vi "Write Pin.vi"(0 "NXP in":refnum<class "NXP.lvclass">, 5 "VISA resource name":refnum<visa-resource-name>, 7 "Pin":u16, 9 "Port 3":u16, 11 "error in (no error)":errorcluster, 12 "Set Pin":bool) -> (4 "NXP out":refnum<class "NXP.lvclass">, 6 "VISA resource name 2":refnum<visa-resource-name>, 15 "error out":errorcluster)   [LabVIEW 2020, in "NXP.lvclass"]
uses:
  NXP.lvclass
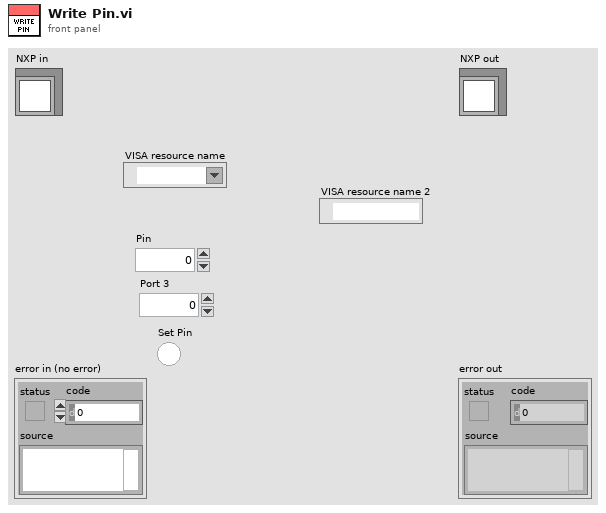
[diagram p1: front panel]
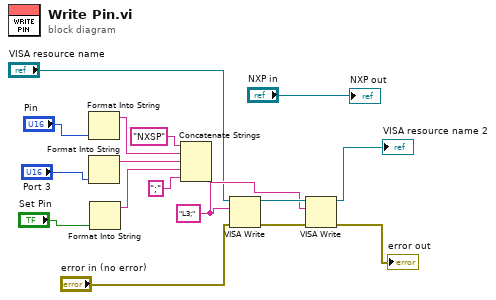
[diagram p0: block diagram]
diagram:
  w12 = "L3;" ("write buffer")
  n1 = Format Into String("Pin") -> (resulting string=w15:string)  [unwired: 3 in, 1 out]
  n2 = Format Into String("Port 3") -> (resulting string=w14:string)  [unwired: 3 in, 1 out]
  n3 = Format Into String("Set Pin") -> (resulting string=w6:string)  [unwired: 3 in, 1 out]
  n4 = Concatenate Strings("NXSP" ("string"), w15, w14, w6, ";" ("string")) -> ()  [unwired: 1 out]
  n5 = VISA Write(VISA resource name="VISA resource name", write buffer=w12, error in (no error)="error in (no error)") -> (VISA resource name out=w13:refnum<visa-resource-name>, error out=w11:errorcluster)  [unwired: 1 out]
  n6 = VISA Write(VISA resource name=w13, write buffer=w12, error in (no error)=w11) -> (VISA resource name out=→"VISA resource name 2":refnum<visa-resource-name>, error out=→"error out":errorcluster)  [unwired: 1 out]
  "NXP out" <- "NXP in"
